vi "SetPosition__slk_mt.vi"(8 "error in (no error)":errorcluster, 11 "label in":refnum<class "Label__slk_mt.lvclass">) -> (0 "error out":errorcluster, 3 "label out":refnum<class "Label__slk_mt.lvclass">)   [LabVIEW 2020, in "Lazyboots Menu Tool.lvlib" / "Label__slk_mt.lvclass"]
doc: "Sets position of label object."
uses:
  Label__slk_mt.lvclass
  Label__slk_mt.lvclass/Label__slk_mt.ctl
  Segment/Segment__slk_mt.lvclass
panel:
  # "SetPosition__slk_mt.vi\nSets position of label object.\n\nNOTICE -- YOU MUST LEAVE THIS NOTICE IN PLACE.\n\nCopyright (c) 2011, LIANG LIU Shawn.Liu.cn@gmail.com\nAll rights reserved.\n\nRedistribution and use in source and binary forms, with or without modification, are permitted provided that the following conditions are met:\n-Redistributions of source code must retain the above copyright notice, this list of conditions and the following disclaimer.\n-Redistributions in binary form must reproduce the above copyright notice, this list of conditions and the following disclaimer in the documentation and/or other materials provided with the distribution.\n-Neither the name of the eLp nor the names of its contributors may be used to endorse or promote products derived from this software without specific prior written permission.\n\nTHIS SOFTWARE IS PROVIDED BY THE COPYRIGHT HOLDERS AND CONTRIBUTORS \"AS IS\" AND ANY EXPRESS OR IMPLIED WARRANTIES, INCLUDING, BUT NOT LIMITED TO, THE IMPLIED WARRANTIES OF MERCHANTABILITY AND FITNESS FOR A PARTICULAR PURPOSE ARE DISCLAIMED. IN NO EVENT SHALL THE COPYRIGHT HOLDER OR CONTRIBUTORS BE LIABLE FOR ANY DIRECT, INDIRECT, INCIDENTAL, SPECIAL, EXEMPLARY, OR CONSEQUENTIAL DAMAGES (INCLUDING, BUT NOT LIMITED TO, PROCUREMENT OF SUBSTITUTE GOODS OR SERVICES; LOSS OF USE, DATA, OR PROFITS; OR BUSINESS INTERRUPTION) HOWEVER CAUSED AND ON ANY THEORY OF LIABILITY, WHETHER IN CONTRACT, STRICT LIABILITY, OR TORT (INCLUDING NEGLIGENCE OR OTHERWISE) ARISING IN ANY WAY OUT OF THE USE OF THIS SOFTWARE, EVEN IF ADVISED OF THE POSSIBILITY OF SUCH DAMAGE."
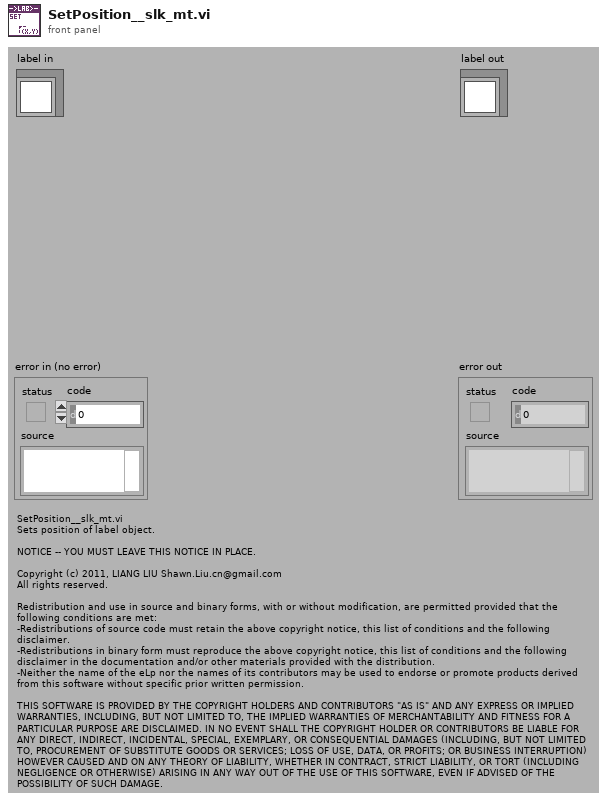
[diagram p1: front panel]
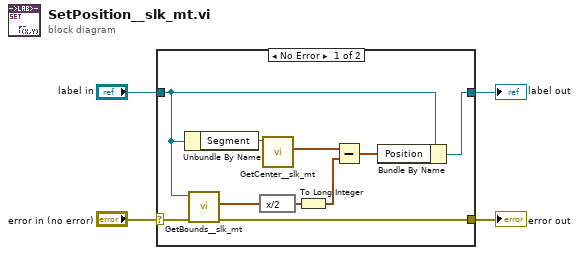
[diagram p0: block diagram]
diagram:
  n1 = case shown="No Error" "error in (no error)" {
    selector: "error in (no error)" -> [w8 w15]
    tunnel: [w7 w15] -> w3
    tunnel: [w14 w16] -> w1
    tunnel: "label in" -> [w6 w16]
    frame No Error {
      n2 = Unbundle By Name(w6) -> ("Segment"=w5:refnum<class "Segment__slk_mt.lvclass">)
      n3 = call "GetBounds__slk_mt.vi"("error in (no error)"=w8, "label in"=w6) -> ("error out"=w7:errorcluster, "bounds"=w9:cluster{"Width":u32, "Height":u32})  [unwired: 7 in, 1 out]
      n4 = expression code="x/2"(w9) -> (w12:cluster{"Width":u32, "Height":u32})
      n5 = call "GetCenter__slk_mt.vi"("segment in"=w5) -> ("center"=w13:cluster{"X":i32, "Y":i32})  [unwired: 8 in, 2 out]
      n6 = To Long Integer(number=w12) -> (32bit integer=w11:cluster{"Width":i32, "Height":i32})
      n7 = Subtract(x=w13, y=w11) -> (x-y=w10:cluster{i32, i32})
      n8 = Bundle By Name(cluster=w6, "Position"=w10) -> (w14:refnum<class "Label__slk_mt.lvclass">)
    }
    frame Error {
    }
  }
  "error out" <- w3
  "label out" <- w1
